vi "unload.vi"(8 "error in (no error)":errorcluster, 10 "imt_testsys_reg_event":T1, 11 "imt_testsys_event":T2) -> (0 "error out":errorcluster)   [LabVIEW 2015, in "pdbm_test_system.lvlib"]
uses:
  pdbm_test_system.lvlib
  pdbm_testsys_taskroute_inter/UsrDefine/pdbm_testsys_reqst_data.ctl
  UsrDefine/pdbm_testsystem_feedback_data.ctl
  pdbm_testsys_taskroute_inter/pdbm_testsys_taskroute_inter.lvlib
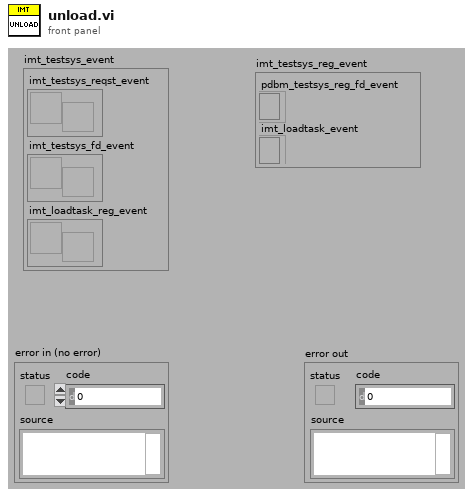
[diagram p1: front panel]
types:
  T1 = cluster{"pdbm_testsys_reg_fd_event":refnum<event-registration>, "imt_loadtask_event":refnum<event-registration>}
  T2 = cluster{"imt_testsys_reqst_event":refnum<user-event>, "imt_testsys_fd_event":refnum<user-event>, "imt_loadtask_reg_event":refnum<user-event>}
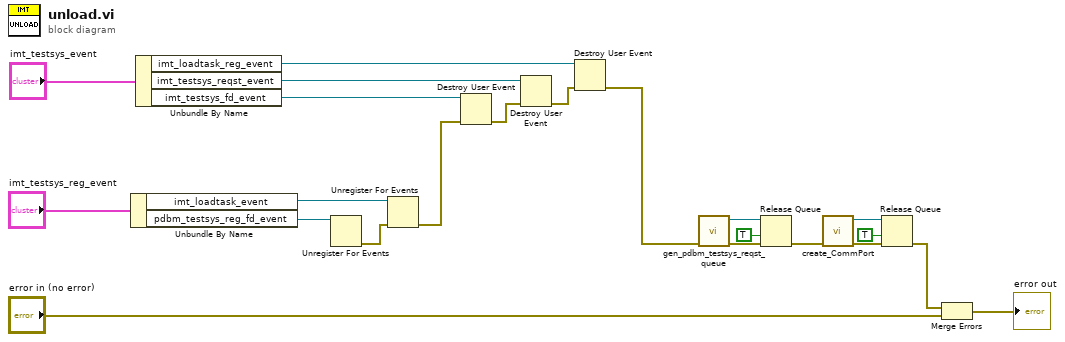
[diagram p0: block diagram]
diagram:
  n1 = Unbundle By Name("imt_testsys_reg_event") -> ("imt_loadtask_event"=w6:refnum<event-registration>, "pdbm_testsys_reg_fd_event"=w21:refnum<event-registration>)
  n2 = Unbundle By Name("imt_testsys_event") -> ("imt_loadtask_reg_event"=w3:refnum<user-event>, "imt_testsys_reqst_event"=w18:refnum<user-event>, "imt_testsys_fd_event"=w19:refnum<user-event>)
  n3 = Unregister For Events(event registration refnum=w21) -> (error out=w5:errorcluster)  [unwired: 1 in]
  n4 = Unregister For Events(event registration refnum=w6, error in=w5) -> (error out=w4:errorcluster)
  n5 = Destroy User Event(user event=w19, error in=w4) -> (error out=w17:errorcluster)
  n6 = Destroy User Event(user event=w18, error in=w17) -> (error out=w2:errorcluster)
  n7 = Destroy User Event(user event=w3, error in=w2) -> (error out=w1:errorcluster)
  n8 = call "gen_pdbm_testsys_reqst_queue.vi"("error in (no error)"=w1) -> ("error IO"=w15:errorcluster, "pdbm_testsys_reqst_event"=w16:refnum<queue>)  [unwired: 9 in]
  n9 = Release Queue(queue=w16, force destroy? (F)=TRUE, error in (no error)=w15) -> (error out=w13:errorcluster)  [unwired: 2 out]
  n10 = call "create_CommPort.vi"("error in (no error)"=w13) -> ("error out"=w12:errorcluster, "pdbm_testsys_feedback_event"=w11:refnum<queue>)  [unwired: 9 in]
  n11 = Release Queue(queue=w11, force destroy? (F)=TRUE, error in (no error)=w12) -> (error out=w8:errorcluster)  [unwired: 2 out]
  n12 = Merge Errors(w8, "error in (no error)") -> (→"error out":errorcluster)
